vi "Actor Core.vi"(8 "error in":errorcluster, 11 "Nested in":refnum<class "StepMotorController.lvclass">) -> (0 "error out":errorcluster, 3 "Actor out":refnum<class "Actor.lvclass">)   [LabVIEW 2020, in "StepMotorController.lvlib" / "StepMotorController.lvclass"]
doc: "(<B>Filename</B>: Actor Framework.lvlib:Actor.lvclass:Actor Core.vi)\n\nReceives messages to the actor, reacts to them, and initiates any error handling that may shut the actor down.\n\nDescendant classes may override this VI to append parallel tasks for the actor to complete while it handles messages. Overrides use the Call Parent Method node."
uses:
  StepMotorController.lvclass
  C:/Program Files/National Instruments/LabVIEW 2020/vi.lib/ActorFramework/Actor/Actor.lvclass
  <vilib>/ActorFramework/Actor/Actor.lvclass
  StepMotorController.lvclass/StepMotorController.ctl
  <vilib>/ActorFramework/Actor/Actor.lvclass/Actor.ctl
  <vilib>/ActorFramework/Message Enqueuer/Message Enqueuer.lvclass/Message Enqueuer.ctl
  Model/Hardware Abstraction Layer/Component/Stage/Stage Messages/SetRelativePositionUm Msg/SetRelativePositionUm Msg.lvclass/SetRelativePositionUm Msg.ctl
  <vilib>/ActorFramework/Message Enqueuer/Init from Existing Queue.vi
  <vilib>/ActorFramework/Message Enqueuer/Enqueue.vi
  <vilib>/ActorFramework/Stop Msg/Stop Msg.lvclass
  C:/Program Files/National Instruments/LabVIEW 2020/vi.lib/ActorFramework/Message/Message.lvclass
  Model/Hardware Abstraction Layer/Component/Stage/Stage Messages/SetRelativePositionUm Msg/SetRelativePositionUm Msg.lvclass
  Model/Hardware Abstraction Layer/Component/Stage/Stage Messages/Home Msg/Home Msg.lvclass
  <vilib>/ActorFramework/Message Priority Queue/Priority Enqueue.vi
  <vilib>/ActorFramework/Message Enqueuer/Message Enqueuer.lvclass
panel:
  in  "TIR Position":dbl min=-999999.0 max=999999.0
  in  "FindEPI":bool
  out "EPILimit":bool
  out "TIRFLimit":bool
  in  "MicroStage+":dbl min=0.0 max=5000.0
  in  "EPI+":bool
  in  "EPI++":bool
  in  "TIRF++":bool
  in  "TIRF+":bool
  out "TirfModuleScollBar":i16(slide) scale=-20000.0..20000.0
  # "TIRF"
  # "EPI"
  # "Inc."
  # "um"
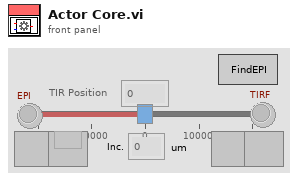
[diagram p1: front panel]
types:
  T1 = cluster{"Stop":refnum<user-event>, "TirfModuleScollBar":refnum<user-event>, "TIRFLimit":refnum<user-event>, "EPILimit":refnum<user-event>}
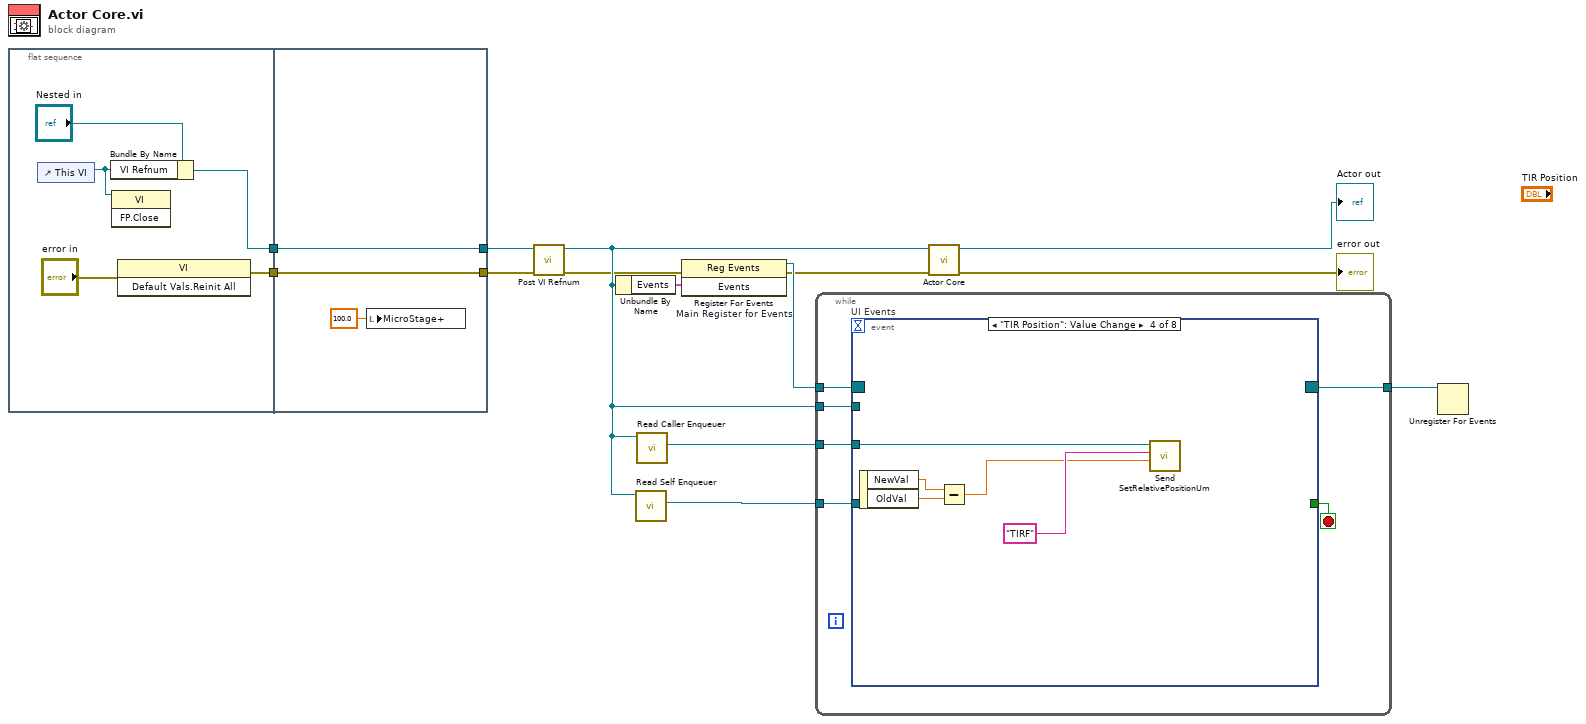
[diagram p0: block diagram]
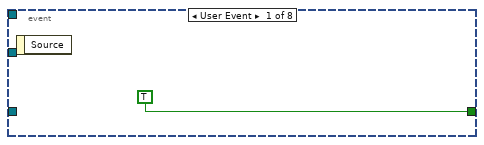
[diagram p2: hidden frame]
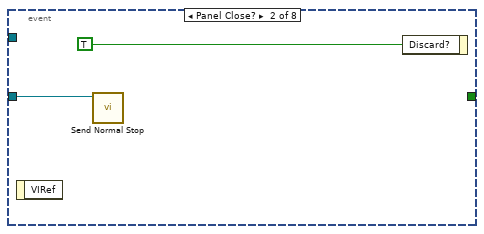
[diagram p3: hidden frame]
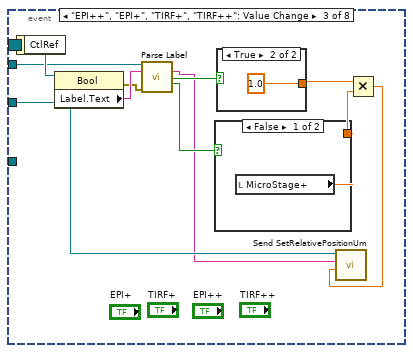
[diagram p4: hidden frame]
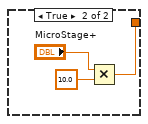
[diagram p5: hidden frame]
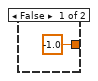
[diagram p6: hidden frame]
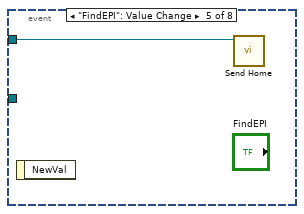
[diagram p7: hidden frame]
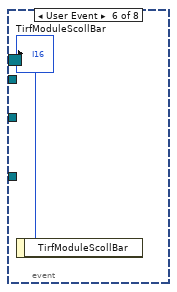
[diagram p8: hidden frame]
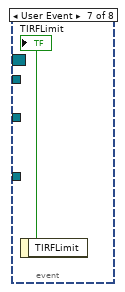
[diagram p9: hidden frame]
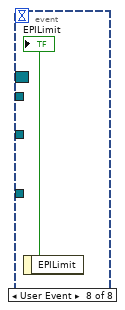
[diagram p10: hidden frame]
diagram:
  n1 = flat-sequence {
    tunnel: [w17] -> w2
    tunnel: [w16] -> w1
    tunnel: [w21] -> w4
    tunnel: [w22] -> w6
    tunnel: w2 -> [w22]
    tunnel: w1 -> [w21]
    frame #0 {
      n2 = control-ref of="This VI"() -> (w15:refnum<vi>)
      n3 = Bundle By Name(cluster="Nested in", "VI Refnum"=w15) -> (w17:refnum<class "StepMotorController.lvclass">)
      n4 = invoke class="VI" method="FP.Close"(reference=w15) -> ()  [unwired: 2 in, 3 out]
      n5 = invoke class="VI" method="Default Vals.Reinit All"(error in="error in") -> (error out=w16:errorcluster)  [unwired: 2 in, 2 out]
    }
    frame #1 {
      n6 = local write "MicroStage+"(100.0 ("MicroStage+")) -> ()
    }
  }
  n7 = call-dynamic "Post VI Refnum.vi"("error in (no error)"=w4, "Stage Controller StepMotor in"=w6) -> ("error out"=w3:errorcluster, "Stage Controller StepMotor out"=w5:refnum<class "StepMotorController.lvclass">)  [unwired: 8 in]
  n8 = Unbundle By Name(w5) -> ("Events"=w11:T1)
  n9 = call <vilib>:"Read Self Enqueuer.vi"("Actor"=w5) -> ("Self Enqueuer"=w9:refnum<class "Message Enqueuer.lvclass">)  [unwired: 10 in]
  n10 = call <vilib>:"Read Caller Enqueuer.vi"("Actor"=w5) -> ("Caller Enqueuer"=w7:refnum<class "Message Enqueuer.lvclass">)  [unwired: 10 in]
  n11 = register-events "Main Register for Events"(error in=w3, w11) -> (reference out=w12:refnum<event-registration>, error out=w8:errorcluster)  [unwired: 1 in]
  n12 = while {
    tunnel: w12 -> [w28]
    tunnel: [w26] -> w10
    tunnel: w9 -> [w25]
    tunnel: w7 -> [w24]
    tunnel: w5 -> [w23]
    stop <- w27 stop-if-true
    n13 = event "UI Events" shown="[3] \"TIR Position\": Value Change" {
      selector: w28 -> [_ _ _ _ _ _ _ _]
      dyn-events: [_ _ _ _ _ _ _ _] -> w26
      timeout: _ -> [_ _ _ _ _ _ _ _]
      tunnel: [TRUE _ _ _ _ _ _ _] -> w27
      tunnel: w25 -> [_ w30 _ _ _ _ _ _]
      tunnel: w24 -> [_ _ w34 w52 w54 _ _ _]
      tunnel: w23 -> [_ _ w41 _ _ _ _ _]
      event User Event {
        n14 = event-data() -> ()  [unwired: 1 in, 1 out]
      }
      event Panel Close? {
        n15 = event-data() -> ()  [unwired: 1 in, 1 out]
        n16 = call <vilib>:"Send Normal Stop.vi"("Message Enqueuer"=w30) -> ()  [unwired: 10 in, 1 out]
        n17 = event-data("Discard?"=TRUE) -> ()  [unwired: 1 in, 1 out]
      }
      event "EPI++", "EPI+", "TIRF+", "TIRF++": Value Change {
        n18 = event-data() -> ("CtlRef"=w42:refnum<vi>)  [unwired: 1 in]
        n19 = property class="Bool"(reference=w42) -> (error out=w39:errorcluster, "Label.Text"=w40:string)  [unwired: 1 in, 1 out]
        n20 = call-dynamic "Parse Label.vi"("Stage Controller StepMotor in"=w41, "Label.Text"=w40, "error in (no error)"=w39) -> ("Stage Label"=w32:string, "Increase?"=w38:bool, "Big Step?"=w37:bool)  [unwired: 8 in, 2 out]
        n21 = case shown="False" w37 {
          tunnel: [w43 w44] -> w35
          frame False {
            n22 = local read "MicroStage+"() -> (w43:dbl)
          }
          frame True {
            n23 = Multiply(x="MicroStage+", y=10.0) -> (x*y=w44:dbl)
          }
        }
        n24 = case shown="True" w38 {
          tunnel: [-1.0 ("XYIncreatement+") 1.0 ("XYIncreatement+")] -> w36
          frame False {
          }
          frame True {
          }
        }
        n25 = Multiply(x=w36, y=w35) -> (x*y=w33:dbl)
        n26 = call "Send SetRelativePositionUm.vi"("RelativeMoveum"=w33, "Stage Label"=w32, "Message Enqueuer"=w34) -> ()  [unwired: 7 in, 2 out]
      }
      event "TIR Position": Value Change {
        n27 = event-data() -> ("NewVal"=w51:dbl, "OldVal"=w50:dbl)  [unwired: 1 in]
        n28 = Subtract(x=w51, y=w50) -> (x-y=w49:dbl)
        n29 = call "Send SetRelativePositionUm.vi"("RelativeMoveum"=w49, "Stage Label"="TIRF", "Message Enqueuer"=w52) -> ()  [unwired: 7 in, 2 out]
      }
      event "FindEPI": Value Change {
        n30 = event-data() -> ()  [unwired: 1 in, 1 out]
        n31 = call "Send Home.vi"("Message Enqueuer"=w54) -> ()  [unwired: 9 in, 2 out]
      }
      event User Event {
        n32 = event-data() -> ("TirfModuleScollBar"=→"TirfModuleScollBar":i16)  [unwired: 1 in]
      }
      event User Event {
        n33 = event-data() -> ("TIRFLimit"=→"TIRFLimit":bool)  [unwired: 1 in]
      }
      event User Event {
        n34 = event-data() -> ("EPILimit"=→"EPILimit":bool)  [unwired: 1 in]
      }
    }
  }
  n35 = call-parent "Actor Core.vi"("error in"=w8, "Actor in"=w5) -> ("error out"=→"error out":errorcluster, "Actor out"=→"Actor out":refnum<class "Actor.lvclass">)  [unwired: 8 in]
  n36 = Unregister For Events(event registration refnum=w10) -> ()  [unwired: 1 in, 1 out]
